vi "Test All.vi"(11 "Error in":errorcluster) -> (15 "Error out":errorcluster)   [LabVIEW 2020, in "StopWatchTests.lvlib"]
doc: "This vi will run all the tests for Stop Watch and a report is generated and stored."
uses:
  StopWatchTests.lvlib
  <vilib>/addons/_JKI Toolkits/Caraya/classes/Test Suite/Define Test Suite (JUnit Report).vi
  <vilib>/addons/_JKI Toolkits/Caraya/classes/Test Suite/Test Suite.lvclass
  <vilib>/addons/_JKI Toolkits/Caraya/classes/Test/Test.lvclass
  <vilib>/Wiresmith Technology/G CLI/CLI Class/CLI.lvclass
panel:
  # "STOP WATCH TEST"
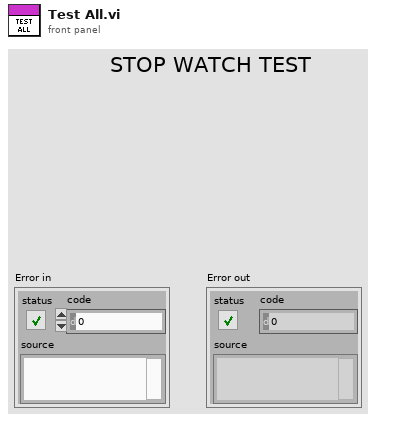
[diagram p1: front panel]
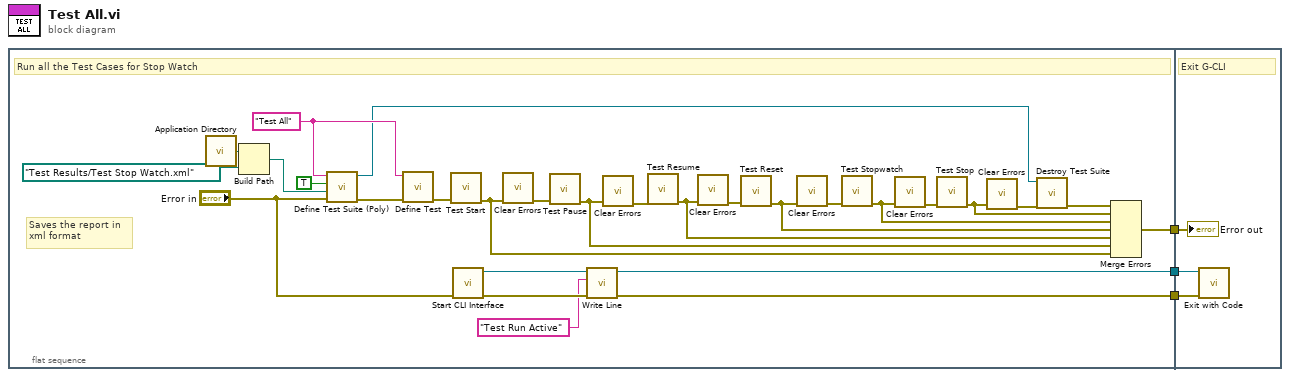
[diagram p0: block diagram]
diagram:
  n1 = flat-sequence {
    tunnel: [w6] -> w3
    tunnel: [w5] -> w2
    tunnel: [w4] -> w1
    tunnel: w3 -> [w34]
    tunnel: w2 -> [w33]
    tunnel: w1 -> [w32]
    frame #0 {
      w27 = "Test All" ("Label (VI Title)")
      # "Saves the report in\nxml format"
      # "Run all the Test Cases for Stop Watch"
      n2 = call <vilib>:"Application Directory.vi"() -> ("Application Directory"=w31:path)
      n3 = Build Path(base path=w31, name or relative path=path "Test Results/Test Stop Watch.xml") -> (appended path=w29:path)
      n4 = call-poly <vilib>:"Define Test Suite (Poly).vi"("error in (no error)"="Error in", "Report Path"=w29, "Interactive"=TRUE, "Label (VI Title)"=w27) -> ("error out"=w26:errorcluster, "Test Suite"=w12:refnum<class "Test Suite.lvclass">)  [unwired: 6 in]
      n5 = call <vilib>:"Define Test.vi"("error in (no error)"=w26, "Label (VI Title)"=w27) -> ("error out"=w25:errorcluster)  [unwired: 9 in]
      n6 = call "Test Start.vi"("Error in"=w25) -> ("Error out"=w22:errorcluster)  [unwired: 14 in]
      n7 = call <vilib>:"Start CLI Interface.vi"("error in (no error)"="Error in") -> ("error out"=w10:errorcluster, "CLI out"=w8:refnum<class "CLI.lvclass">)  [unwired: 7 in, 2 out]
      n8 = call <vilib>:"Clear Errors.vi"("error in (no error)"=w22) -> ("error out"=w24:errorcluster)  [unwired: 5 in, 1 out]
      n9 = call "Test Pause.vi"("Error in"=w24) -> ("Error out"=w21:errorcluster)  [unwired: 14 in]
      n10 = call <vilib>:"Write Line.vi"("error in (no error)"=w10, "Text to Write"="Test Run Active", "CLI in"=w8) -> ("error out"=w5:errorcluster, "CLI out"=w4:refnum<class "CLI.lvclass">)  [unwired: 7 in]
      n11 = call <vilib>:"Clear Errors.vi"("error in (no error)"=w21) -> ("error out"=w23:errorcluster)  [unwired: 5 in, 1 out]
      n12 = call "Test Resume.vi"("Error in"=w23) -> ("Error out"=w20:errorcluster)  [unwired: 14 in]
      n13 = call <vilib>:"Clear Errors.vi"("error in (no error)"=w20) -> ("error out"=w18:errorcluster)  [unwired: 5 in, 1 out]
      n14 = call "Test Reset.vi"("Error in"=w18) -> ("Error out"=w17:errorcluster)  [unwired: 14 in]
      n15 = call <vilib>:"Clear Errors.vi"("error in (no error)"=w17) -> ("error out"=w19:errorcluster)  [unwired: 5 in, 1 out]
      n16 = call "Test Stopwatch.vi"("Error in"=w19) -> ("Error out"=w15:errorcluster)  [unwired: 14 in]
      n17 = call <vilib>:"Clear Errors.vi"("error in (no error)"=w15) -> ("error out"=w16:errorcluster)  [unwired: 5 in, 1 out]
      n18 = call "Test Stop.vi"("Error in"=w16) -> ("Error out"=w14:errorcluster)  [unwired: 14 in]
      n19 = call <vilib>:"Clear Errors.vi"("error in (no error)"=w14) -> ("error out"=w13:errorcluster)  [unwired: 5 in, 1 out]
      n20 = call-dynamic "Destroy Test Suite.vi"("error in (no error)"=w13, "Test Suite in"=w12) -> ("error out"=w7:errorcluster)  [unwired: 8 in, 1 out]
      n21 = Merge Errors(w7, w14, w15, w17, w20, w21, w22) -> (w6:errorcluster)
    }
    frame #1 {
      # "Exit G-CLI"
      n22 = call <vilib>:"Exit with Code.vi"("error in (no error)"=w33, "CLI in"=w32) -> ()  [unwired: 9 in, 1 out]
      "Error out" <- w34
    }
  }
